vi "DPT Panel RMC Calculator.vi"(0 "Scale Com Port":refnum<visa-resource-name>="COM1", 5 "Bone Dry Weight (lbs)":T2 format="%.3f", 7 "Read Scale Weight":bool, 11 "Error In":errorcluster) -> (6 "DPT IMC Data Out":T3={"Measured IMC (lbs)"=7.0, "Actual Initial RMC (%)"=7.0, "RMC (Desired %)"=100.0, "Bone Dry Wt(lbs)"=7.0, "Tolerance(%)"=5.0, "Actual Final RMC (%)"=7.0, "CEF (lbf/kWh)"=0.0, "Minimum Weight (lbf)"=0.0, "Average Weight (lbf)"=0.0, "Maximum Weight (lbf)"=0.0, "Measured IMC In Range?"=FALSE, "Moisture Reduction Factor"=55.5, "Field Use Factor"=1.04, "Empty Dryer Cold Weigth"=0.0, "Energy Standard"=enum."D2-Automatic Dryer", "Weight Cloth (lbs)"=0.0, "Relative Moisture Content (%)"=0.0, "Relative Moisture Content - Avg (%)"=0.0} {"Maximum Weight (lbf)" format="%03_6g"; "Average Weight (lbf)" format="%03_6g"; "Minimum Weight (lbf)" format="%03_6g"; "CEF (lbf/kWh)" format="%03_6g"; "Actual Final RMC (%)" format="%03_6g"; "Tolerance(%)" format="%0#_6g"; "Bone Dry Wt(lbs)" format="%03_6g"; "RMC (Desired %)" format="%0#_6g"; "Actual Initial RMC (%)" format="%03_6g"; "Measured IMC (lbs)" format="%0#_6g"}, 15 "Error Out":errorcluster)   [LabVIEW 2016, in "File Setup.lvlib"]
uses:
  File Setup.lvlib
  Type Definition/DPT IMC Data.ctl
  Washer DOE/Type Definitions/DOE Dryer Standard.ctl
  Custom Pallet Controls/Custom Pallet DBL.ctl
  Custom Pallet Controls/Custom Pallet Forward.ctl
panel:
  in  "Complete":T1
  out "Average Weight (lbs)":T2 format="%.3f"
  out "Maximum Weight (lbs)":T2 format="%.3f"
  out "Minimum Weight (lbs)":T2 format="%.3f"
  in  "Relative Moisture Content (Desired)":T2 format="%.3f"
  in  "Tolerance %":T2=5.0 format="%.3f"
  in  "Tab Control":enum32{"Page 1", "Page 2"}(tab)
  out "Actual Relative Moisture Content (%)":T2 format="%.2f"
  in  "Measured Initial Moisture Content (lbs)":T2 format="%.3f"
  # "RMC Calculator"
  # "Calculated Result"
  # "User Input"
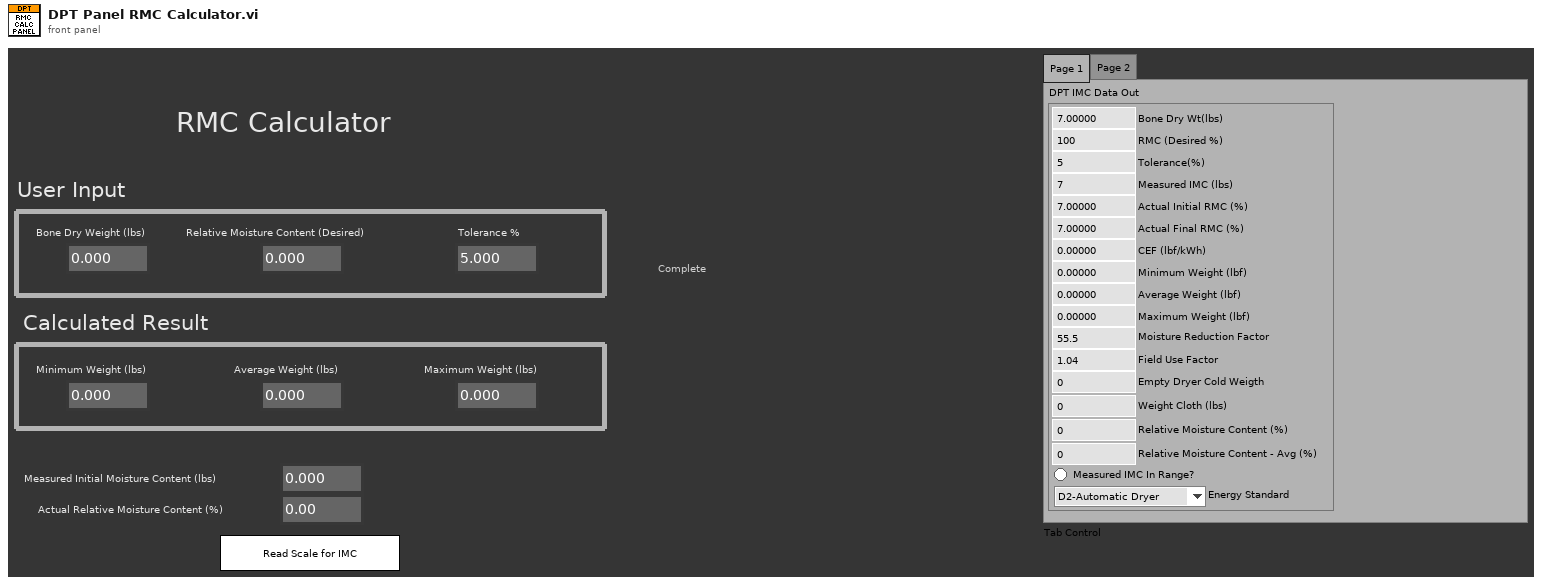
[diagram p1: front panel]
types:
  T1 = typedef "Custom Pallet Forward.ctl" = bool
  T2 = typedef "Custom Pallet DBL.ctl" = dbl
  T3 = typedef "DPT IMC Data.ctl" = cluster{"Measured IMC (lbs)":dbl, "Actual Initial RMC (%)":dbl, "RMC (Desired %)":dbl, "Bone Dry Wt(lbs)":dbl, "Tolerance(%)":dbl, "Actual Final RMC (%)":dbl, "CEF (lbf/kWh)":dbl, "Minimum Weight (lbf)":dbl, "Average Weight (lbf)":dbl, "Maximum Weight (lbf)":dbl, "Measured IMC In Range?":bool, "Moisture Reduction Factor":dbl, "Field Use Factor":dbl, "Empty Dryer Cold Weigth":dbl, "Energy Standard":T4, "Weight Cloth (lbs)":dbl, "Relative Moisture Content (%)":dbl, "Relative Moisture Content - Avg (%)":dbl}
  T4 = typedef "DOE Dryer Standard.ctl" = enum16{"D2-Automatic Dryer", "D2-Timer Dryer", "D1-Automatic Dryer", "D1-Timer Dryer", "Other"}
  T5 = enum32{"invalid app kind", "Development System", "Run Time System", "Student Edition", "Embedded LabVIEW", "Evaluation", "Custom"}
  T6 = enum32{"Invalid", "Standard", "Closed", "Hidden", "Minimized", "Maximized"}
  T7 = cluster{"Core":cluster{"Current VI Reference":refnum<vi>, "Close Panel on Exit?":bool}, "Average Weight (lbs) Show":T2, "Minimum Weight (lbs) Show":T2, "Maximum Weight (lbs) Show":T2, "Scale Com Port":refnum<visa-resource-name>, "DPT IMC Data":T3}
  T8 = cluster{"Current VI Reference":refnum<vi>, "Close Panel on Exit?":bool}
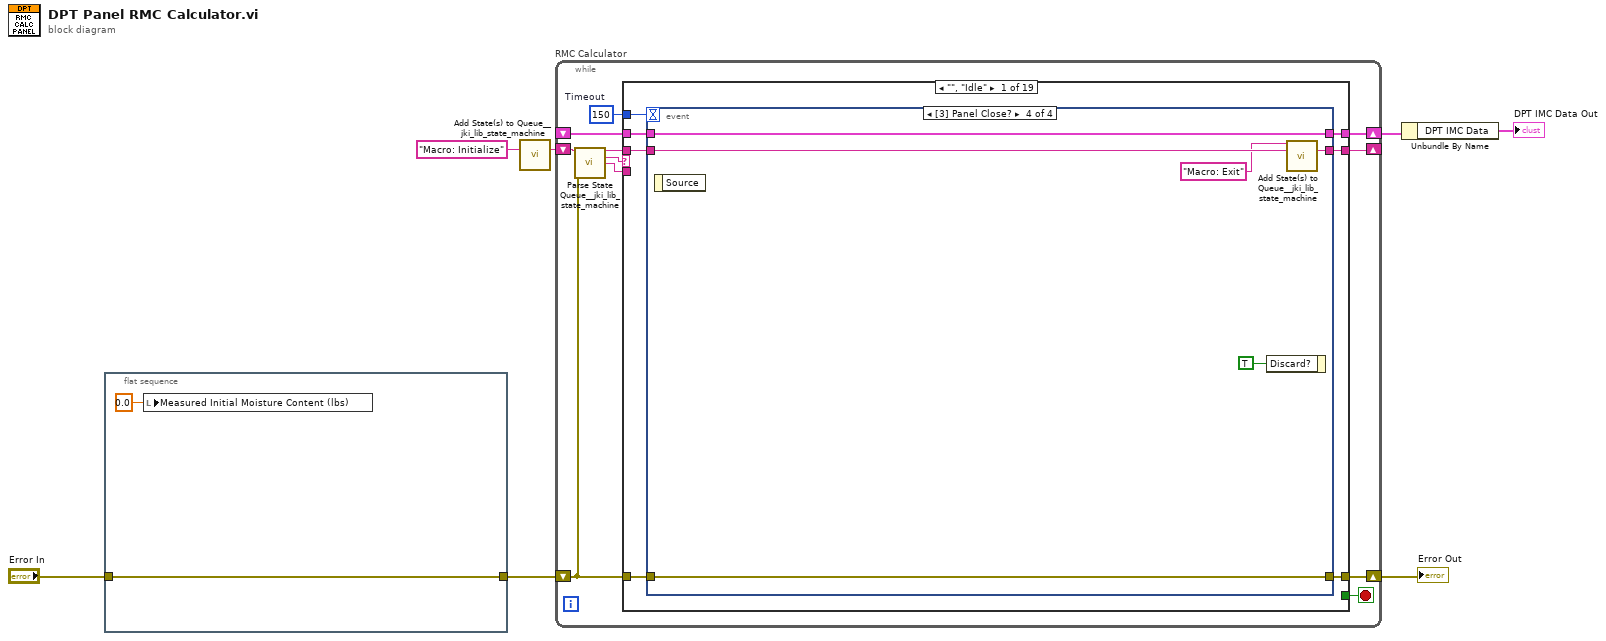
[diagram p0: block diagram]
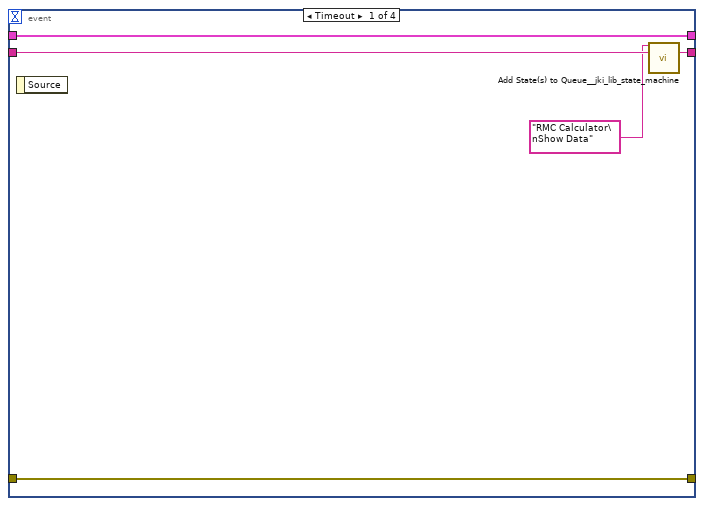
[diagram p2: hidden frame]
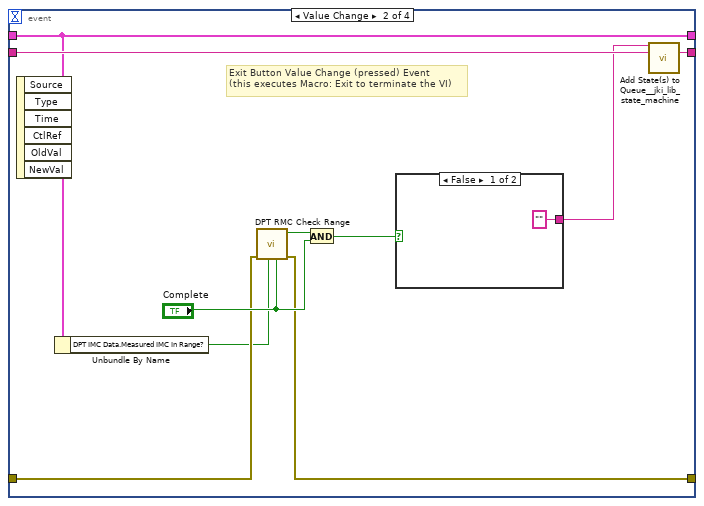
[diagram p3: hidden frame]
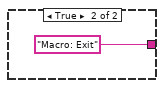
[diagram p4: hidden frame]
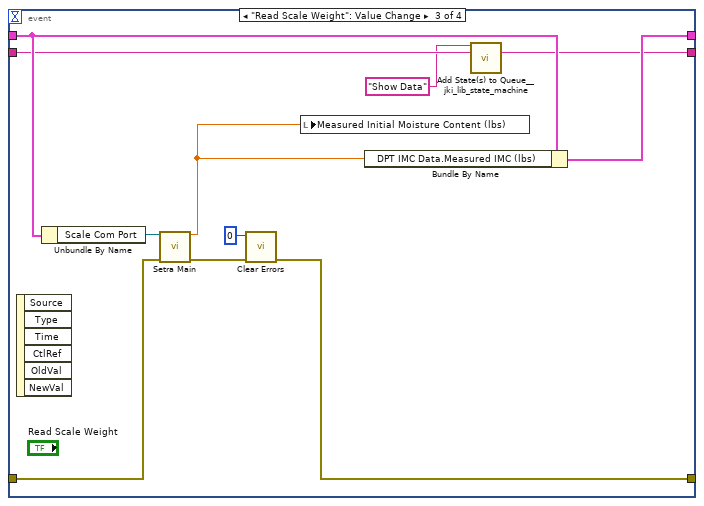
[diagram p5: hidden frame]
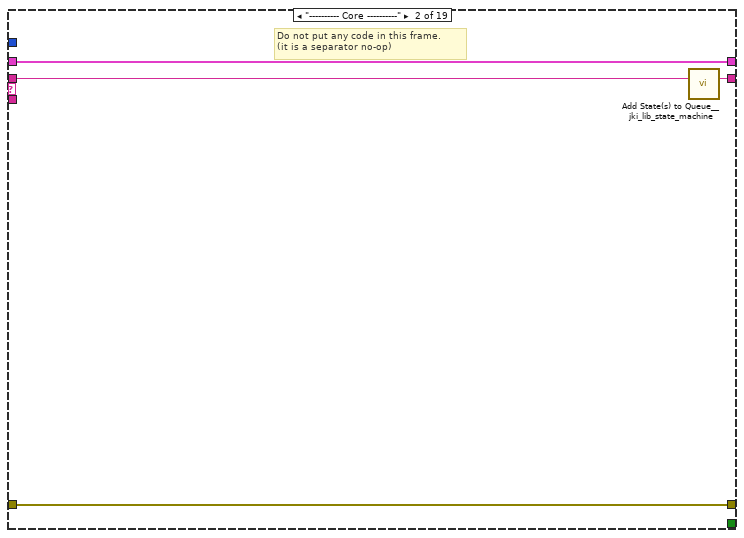
[diagram p6: hidden frame]
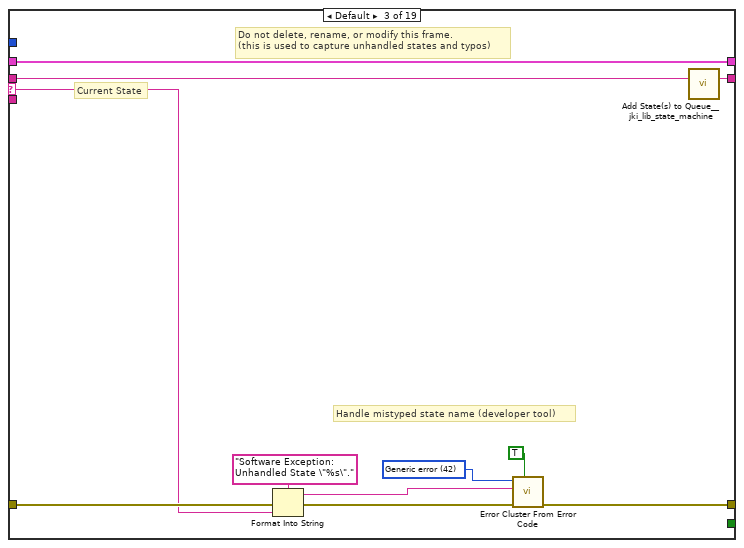
[diagram p7: hidden frame]
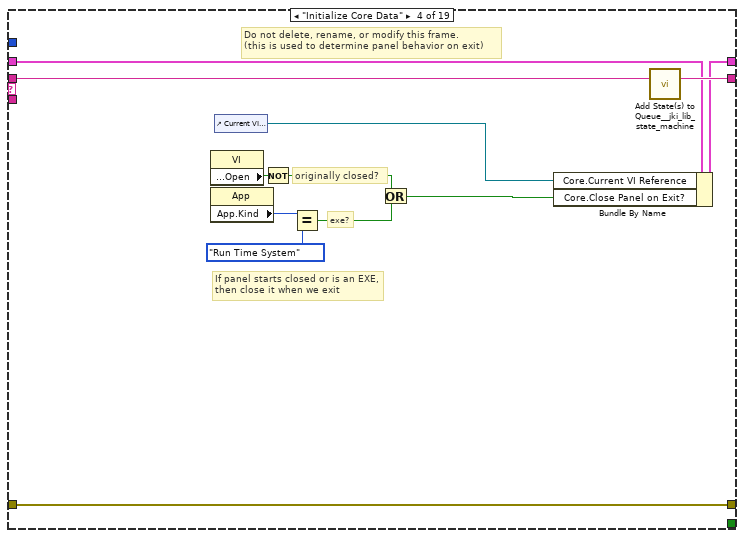
[diagram p8: hidden frame]
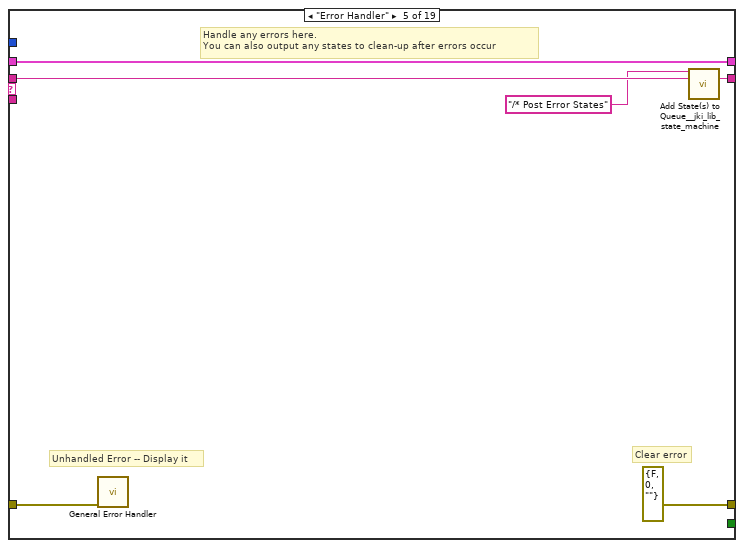
[diagram p9: hidden frame]
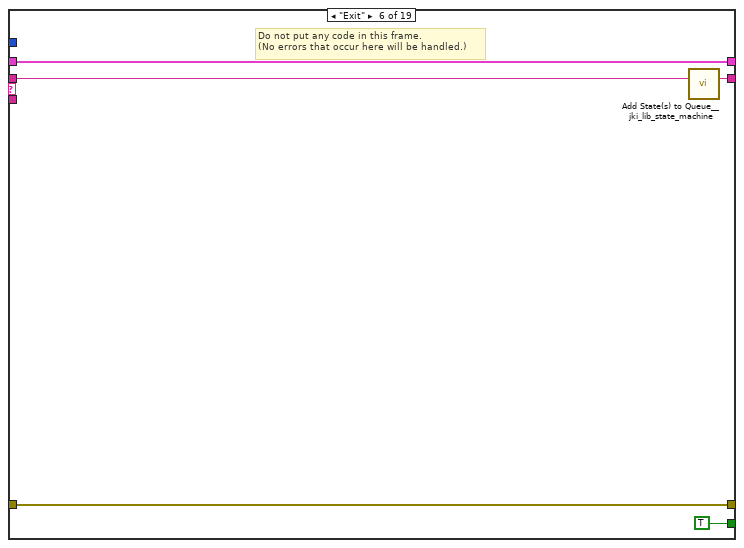
[diagram p10: hidden frame]
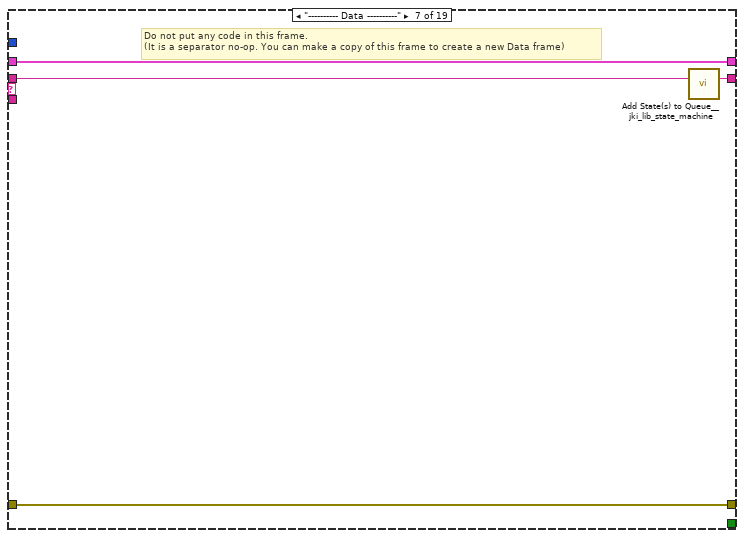
[diagram p11: hidden frame]
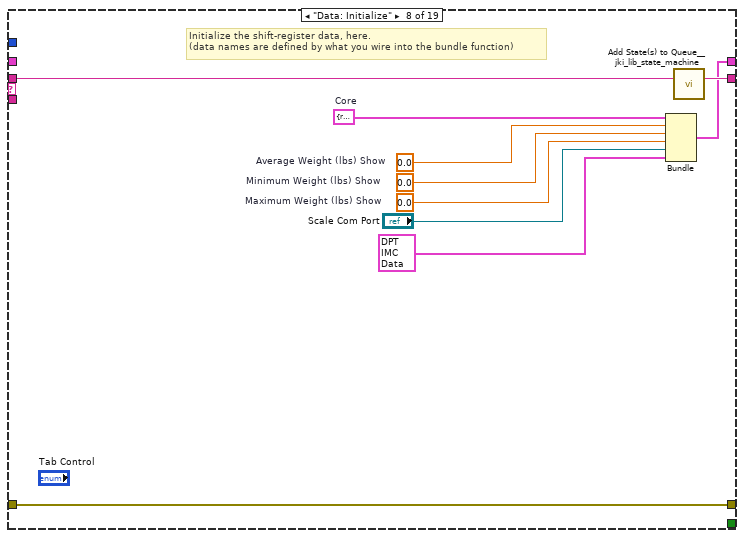
[diagram p12: hidden frame]
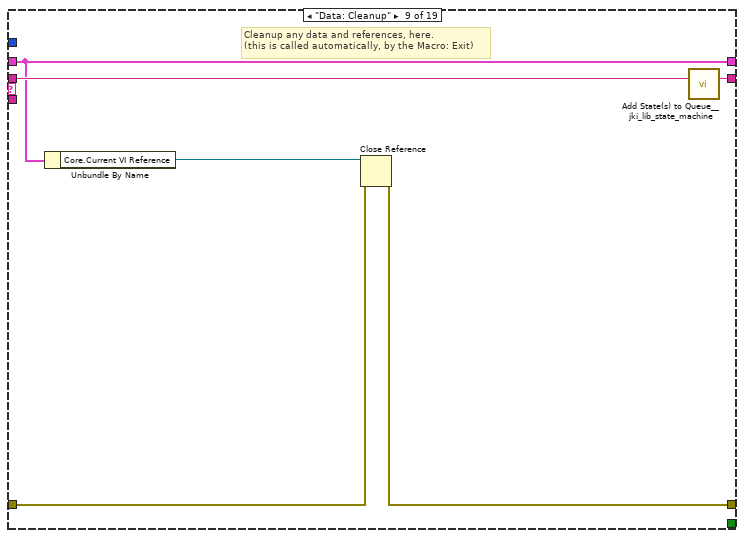
[diagram p13: hidden frame]
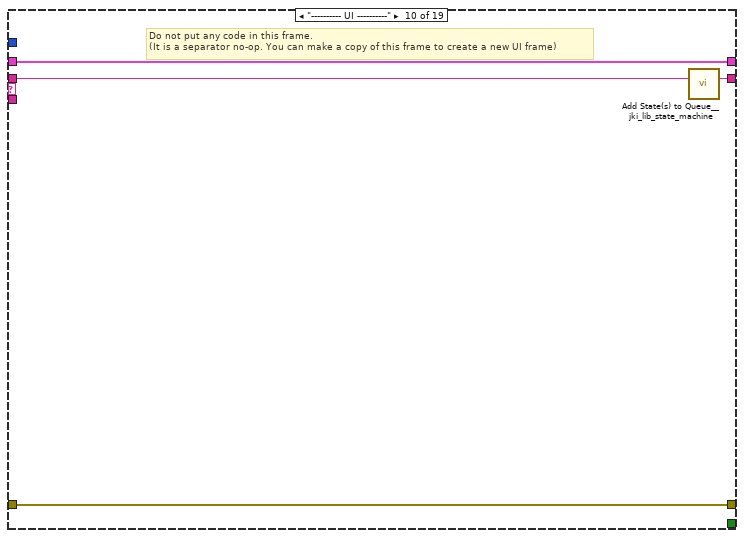
[diagram p14: hidden frame]
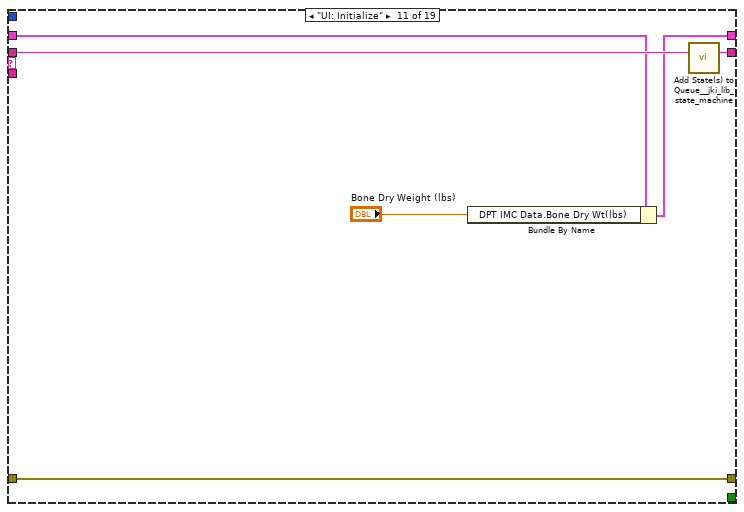
[diagram p15: hidden frame]
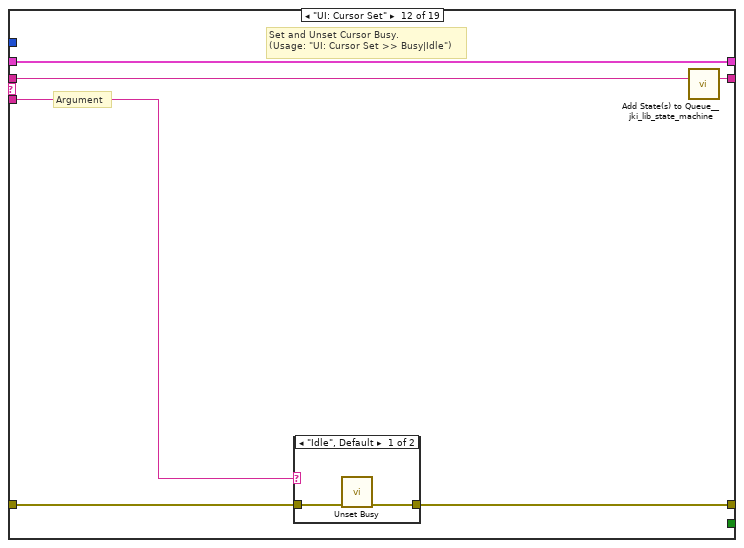
[diagram p16: hidden frame]
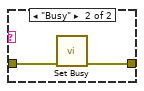
[diagram p17: hidden frame]
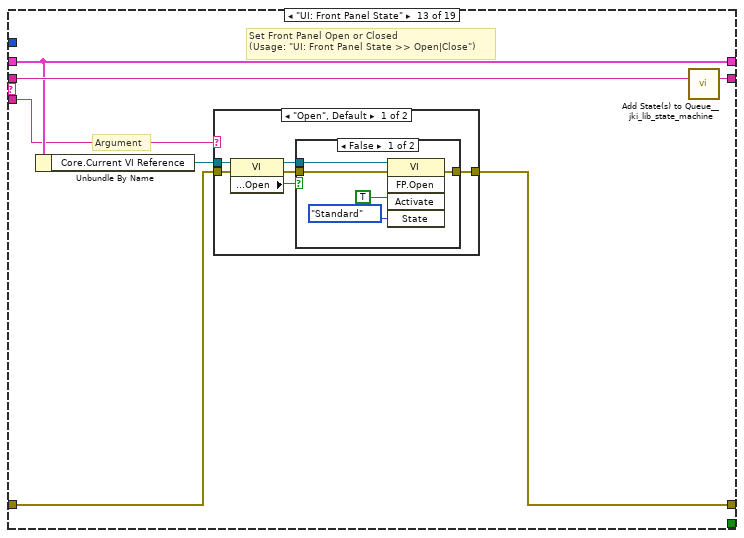
[diagram p18: hidden frame]
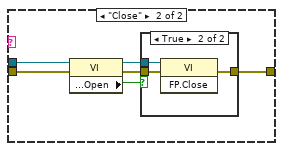
[diagram p20: hidden frame]
diagram:
  n1 = flat-sequence {
    tunnel: "Error In" -> [w8]
    tunnel: [w8] -> w3
    frame #0 {
      n2 = local write "Measured Initial Moisture Content (lbs)"(0.0 ("Measured IMC(Initial Moisture Content)")) -> ()
    }
  }
  n3 = call <vilib>:"Add State(s) to Queue__jki_lib_state_machine.vi"("State(s) in (\"\")"="Macro: Initialize") -> ("States Out"=w7:string)  [unwired: 14 in]
  n4 = while "RMC Calculator" {
    shift-right: [w13] -> w2
    shift-left: _ -> [w12]
    shift-right: [w16] -> w5
    shift-left: w3 -> [w10]
    shift-right: [w15] -> _
    shift-left: w7 -> [w17]
    stop <- w14 stop-if-true
    w11 = 150  # Timeout
    n5 = call <vilib>:"Parse State Queue__jki_lib_state_machine.vi"("State Queue"=w17, "Error In (no error)"=w10) -> ("Remaining States"=w19:string, "Current State"=w20:string, "Arguments"=w18:string)  [unwired: 11 in]
    n6 = case shown="\"\", \"Idle\"" w20 {
      selector: w20 -> [_ _ w66 _ _ _ _ _ _ _ _ _ _ _ _ _ _ _ _]
      tunnel: w19 -> [w27 w65 w70 w88 w94 w99 w103 w113 w119 w123 w129 w135 w146 w172 w177 w187 w191 w199 w209]
      tunnel: w18 -> [_ _ _ _ _ _ _ _ _ _ _ w130 w140 _ _ _ _ _ _]
      tunnel: w12 -> [w25 w62 w68 w79 w91 w97 w100 _ w114 w120 w126 w133 w142 w169 w174 w184 w188 w193 w206]
      tunnel: [w24 w63 w72 w85 errorcluster {"status"=FALSE, "code"=0, "source"=""} ("error out") w96 w101 w110 w115 w121 w127 w131 w143 w170 w175 w185 w189 w197 w207] -> w16
      tunnel: w10 -> [w23 w63 w71 w85 w90 w96 w101 w110 w116 w121 w127 w132 w144 w170 w175 w185 w189 w196 w207]
      tunnel: [w26 w64 w69 w87 w93 w98 w102 w112 w118 w122 w128 w134 w145 w171 w176 w186 w190 w198 w208] -> w15
      tunnel: [_ _ _ _ _ TRUE _ _ _ _ _ _ _ _ _ _ _ _ _] -> w14
      tunnel: [w22 w62 w68 w86 w91 w97 w100 w111 w114 w120 w125 w133 w142 w169 w174 w184 w188 w195 w206] -> w13
      tunnel: w11 -> [w21 _ _ _ _ _ _ _ _ _ _ _ _ _ _ _ _ _ _]
      frame "", "Idle" {
        n7 = event shown="[3] Panel Close?" {
          selector: _ -> [_ _ _ _]
          dyn-events: _ -> [_ _ _ _]
          timeout: w21 -> [_ _ _ _]
          tunnel: w27 -> [w32 w42 w51 w61]
          tunnel: [w31 w41 w50 w60] -> w26
          tunnel: w25 -> [w29 w34 w53 w58]
          tunnel: [w30 w36 w47 w59] -> w24
          tunnel: w23 -> [w30 w37 w55 w59]
          tunnel: [w29 w34 w54 w58] -> w22
          event Timeout {
            n8 = event-data() -> ()  [unwired: 1 in, 1 out]
            n9 = call <vilib>:"Add State(s) to Queue__jki_lib_state_machine.vi"("State(s) in Front (\"\")"="RMC Calculator\nShow Data", "State(s) in (\"\")"=w32) -> ("States Out"=w31:string)  [unwired: 13 in]
          }
          event Value Change {
            # "Exit Button Value Change (pressed) Event\n(this executes Macro: Exit to terminate the VI)"
            n10 = event-data() -> ()  [unwired: 1 in, 6 out]
            n11 = Unbundle By Name(w34) -> ("DPT IMC Data.Measured IMC In Range?"=w33:bool)
            n12 = call "DPT RMC Check Range.vi"("Complete"="Complete", "In Range?"=w33, "Error In"=w37) -> ("Error Out"=w36:errorcluster, "End"=w38:bool)  [unwired: 7 in]
            n13 = And(x=w38, y="Complete") -> (x .and. y?=w35:T1)
            n14 = case shown="False" w35 {
              tunnel: ["" "Macro: Exit"] -> w40
              frame False {
              }
              frame True {
              }
            }
            n15 = call <vilib>:"Add State(s) to Queue__jki_lib_state_machine.vi"("State(s) in Front (\"\")"=w40, "State(s) in (\"\")"=w42) -> ("States Out"=w41:string)  [unwired: 13 in]
          }
          event "Read Scale Weight": Value Change {
            n16 = event-data() -> ()  [unwired: 1 in, 6 out]
            n17 = Unbundle By Name(w53) -> ("Scale Com Port"=w52:refnum<visa-resource-name>)
            n18 = call "Setra Main.vi"("VISA resource name"=w52, "Error In"=w55) -> ("Weight Output"=w45:dbl, "Error Out"=w48:errorcluster)  [unwired: 11 in, 1 out]
            n19 = call <vilib>:"Clear Errors.vi"("error in (no error)"=w48, "specific error code to clear (0: all)"=0) -> ("error out"=w47:errorcluster)  [unwired: 4 in, 1 out]
            n20 = local write "Measured Initial Moisture Content (lbs)"(w45) -> ()
            n21 = Bundle By Name(cluster=w53, "DPT IMC Data.Measured IMC (lbs)"=w45) -> (w54:T7)
            n22 = call <vilib>:"Add State(s) to Queue__jki_lib_state_machine.vi"("State(s) in Front (\"\")"="Show Data", "State(s) in (\"\")"=w51) -> ("States Out"=w50:string)  [unwired: 13 in]
          }
          event Panel Close? {
            n23 = event-data() -> ()  [unwired: 1 in, 1 out]
            n24 = event-data("Discard?"=TRUE) -> ()  [unwired: 1 in, 1 out]
            n25 = call <vilib>:"Add State(s) to Queue__jki_lib_state_machine.vi"("State(s) in Front (\"\")"="Macro: Exit", "State(s) in (\"\")"=w61) -> ("States Out"=w60:string)  [unwired: 13 in]
          }
        }
      }
      frame "---------- Core ----------" {
        # "Do not put any code in this frame.\n(it is a separator no-op)"
        n26 = call <vilib>:"Add State(s) to Queue__jki_lib_state_machine.vi"("State(s) in (\"\")"=w65) -> ("States Out"=w64:string)  [unwired: 14 in]
      }
      frame Default {
        w75 = 42 items=["No error", "Argument error", "Memory is full", "Out of zone", "End of file", "File already open", "Generic file I/O error", "File not found", "File permission error", "Disk is full", "Duplicate path", "Too many files open", "System feature not enabled", "Resource file not found", "Cannot add resource", "Resource not found", "Image not found", "Image memory error", "Pen does not exist", "Config type invalid", "Config token not found", "Config parse error", "Config memory error", "Bad external code format", "Bad external code offset", "External code not present", "Null window", "Destroy window error", "Null menu", "Print aborted", "Bad print record", "Print driver error", "Windows error during printing", "Memory error during printing", "Print dialog error", "Generic print error", "Invalid device refnum", "Device not found", "Device parameter error", "Device unit error", "Cannot open device", "Device call aborted", "Generic error", "Cancelled by user", "Object ID too low", "Object ID too high", "Object not in heap", "Unknown heap", "Unknown object (invalid DefProc)", "Unknown object (DefProc not in table)", "Message out of range", "Invalid (null) method", "Unknown message", "Manager call not supported", "Bad address", "Network operation in progress", "Network operation timed out", "Connection is busy", "Network attribute not supported", "Network error", "Address in use", "System out of memory", "Connection aborted", "Connection refused", "Not connected", "Already connected", "Connection closed", "Initialization error (interapplication manager)", "Bad occurrence", "Wait on unbound occurrence handler", "Occurrence queue overflow", "Datalog type conflict", "Unused", "Unrecognized type (interapplication manager)", "Memory corrupt", "Failed to make temporary DLL", "Old CIN version", "Drag socket not found", "Failed to load drop-object", "Failed to register OLE object", "Failed to release OLE object", "Format specifier type mismatch", "Unknown format specifier", "Too few format specifiers", "Too many format specifiers", "Scan failed", "Newer CIN version", "Error converting to variant", "Runtime menu error", "Password tampered", "Variant attribute not found", "Incompatible variant data type", "Event data is not available", "Event Store is not present", "Occurrence is not found", "Event Queue is not created", "Event info is not available", "Refnum passed is NULL", "Error retrieving Class GUID", "Error retrieving CoClass GUID", "Error retrieving TypeLib GUID.", "Bad built application magic bytes.", "Specific driver is different from the specific driver associated with the Logical Name.", "There is no session opened to the class driver.", "Max Error", "MAX - Error with config objects", "MAX - Error loading configuration", "MAX - Group not supported"]
        # "Current State"
        # "Do not delete, rename, or modify this frame.\n(this is used to capture unhandled states and typos)"
        # "Handle mistyped state name (developer tool)"
        n27 = Format Into String(format string="Software Exception: Unhandled State \"%s\"." ("message"), error in=w71, w66) -> (resulting string=w74:string, error out=w73:errorcluster)  [unwired: 1 in]
        n28 = call <vilib>:"Error Cluster From Error Code.vi"("show call chain? (False)"=TRUE, "error in (no error)"=w73, "error message (\"\")"=w74, "error code (0)"=w75) -> ("error out"=w72:errorcluster)  [unwired: 5 in]
        n29 = call <vilib>:"Add State(s) to Queue__jki_lib_state_machine.vi"("State(s) in (\"\")"=w70) -> ("States Out"=w69:string)  [unwired: 14 in]
      }
      frame "Initialize Core Data" {
        # "Do not delete, rename, or modify this frame.\n(this is used to determine panel behavior on exit)"
        # "originally closed?"
        # "exe?"
        # "If panel starts closed or is an EXE, then close it when we exit"
        n30 = property class="VI"() -> ("Front Panel.Open"=w84:bool)  [unwired: 2 in, 2 out]
        n31 = property class="App"() -> ("App.Kind"=w83:T5)  [unwired: 2 in, 2 out]
        n32 = control-ref of="Current VI Reference"() -> (w77:refnum<vi>)
        n33 = Not(x=w84) -> (.not. x?=w81:bool)
        n34 = Equal?(x=w83, y=T5."Run Time System" ("Application:Kind")) -> (x = y?=w80:bool)
        n35 = Or(x=w81, y=w80) -> (x .or. y?=w78:bool)
        n36 = Bundle By Name(cluster=w79, "Core.Current VI Reference"=w77, "Core.Close Panel on Exit?"=w78) -> (w86:T7)
        n37 = call <vilib>:"Add State(s) to Queue__jki_lib_state_machine.vi"("State(s) in (\"\")"=w88) -> ("States Out"=w87:string)  [unwired: 14 in]
      }
      frame "Error Handler" {
        # "Unhandled Error -- Display it"
        # "Handle any errors here.\nYou can also output any states to clean-up after errors occur"
        # "Clear error"
        n38 = call <vilib>:"General Error Handler.vi"("error in (no error)"=w90) -> ()  [unwired: 10 in, 5 out]
        n39 = call <vilib>:"Add State(s) to Queue__jki_lib_state_machine.vi"("State(s) in Front (\"\")"="/* Post Error States", "State(s) in (\"\")"=w94) -> ("States Out"=w93:string)  [unwired: 13 in]
      }
      frame "Exit" {
        # "Do not put any code in this frame.\n(No errors that occur here will be handled.)"
        n40 = call <vilib>:"Add State(s) to Queue__jki_lib_state_machine.vi"("State(s) in (\"\")"=w99) -> ("States Out"=w98:string)  [unwired: 14 in]
      }
      frame "---------- Data ----------" {
        # "Do not put any code in this frame.\n(It is a separator no-op. You can make a copy of this frame to create a new Data frame)"
        n41 = call <vilib>:"Add State(s) to Queue__jki_lib_state_machine.vi"("State(s) in (\"\")"=w103) -> ("States Out"=w102:string)  [unwired: 14 in]
      }
      frame "Data: Initialize" {
        w106 = T2 0.0  # Maximum Weight (lbs) Show
        w107 = T2 0.0  # Minimum Weight (lbs) Show
        w108 = T2 0.0  # Average Weight (lbs) Show
        w109 = T8 {"Current VI Reference"=refnum, "Close Panel on Exit?"=FALSE}  # Core
        # "Initialize the shift-register data, here.\n(data names are defined by what you wire into the bundle function)"
        n42 = Bundle("Core"=w109, "Average Weight (lbs) Show"=w108, "Minimum Weight (lbs) Show"=w107, "Maximum Weight (lbs) Show"=w106, "Scale Com Port"="Scale Com Port", "DPT IMC Data"=T3 {"Measured IMC (lbs)"=0.0, "Actual Initial RMC (%)"=0.0, "RMC (Desired %)"=0.0, "Bone Dry Wt(lbs)"=0.0, "Tolerance(%)"=5.0, "Actual Final RMC (%)"=7.0, "CEF (lbf/kWh)"=0.0, "Minimum Weight (lbf)"=0.0, "Average Weight (lbf)"=0.0, "Maximum Weight (lbf)"=0.0, "Measured IMC In Range?"=FALSE, "Moisture Reduction Factor"=55.5, "Field Use Factor"=1.04, "Empty Dryer Cold Weigth"=0.0, "Energy Standard"=enum."D2-Automatic Dryer", "Weight Cloth (lbs)"=0.0, "Relative Moisture Content (%)"=0.0, "Relative Moisture Content - Avg (%)"=0.0}) -> (w111:T7)  [unwired: 1 in]
        n43 = call <vilib>:"Add State(s) to Queue__jki_lib_state_machine.vi"("State(s) in (\"\")"=w113) -> ("States Out"=w112:string)  [unwired: 14 in]
      }
      frame "Data: Cleanup" {
        # "Cleanup any data and references, here.\n(this is called automatically, by the Macro: Exit)"
        n44 = Unbundle By Name(w114) -> ("Core.Current VI Reference"=w117:refnum<vi>)
        n45 = Close Reference(reference=w117, error in (no error)=w116) -> (error out=w115:errorcluster)
        n46 = call <vilib>:"Add State(s) to Queue__jki_lib_state_machine.vi"("State(s) in (\"\")"=w119) -> ("States Out"=w118:string)  [unwired: 14 in]
      }
      frame "---------- UI ----------" {
        # "Do not put any code in this frame.\n(It is a separator no-op. You can make a copy of this frame to create a new UI frame)"
        n47 = call <vilib>:"Add State(s) to Queue__jki_lib_state_machine.vi"("State(s) in (\"\")"=w123) -> ("States Out"=w122:string)  [unwired: 14 in]
      }
      frame "UI: Initialize" {
        n48 = Bundle By Name(cluster=w126, "DPT IMC Data.Bone Dry Wt(lbs)"="Bone Dry Weight (lbs)") -> (w125:T7)
        n49 = call <vilib>:"Add State(s) to Queue__jki_lib_state_machine.vi"("State(s) in (\"\")"=w129) -> ("States Out"=w128:string)  [unwired: 14 in]
      }
      frame "UI: Cursor Set" {
        # "Argument"
        # "Set and Unset Cursor Busy.\n(Usage: \"UI: Cursor Set >> Busy|Idle\")"
        n50 = case shown="\"Idle\", Default" w130 {
          tunnel: w132 -> [w137 w139]
          tunnel: [w136 w138] -> w131
          frame "Idle", Default {
            n51 = call <vilib>:"Unset Busy.vi"("error in (no error)"=w137) -> ("error out"=w136:errorcluster)  [unwired: 10 in]
          }
          frame "Busy" {
            n52 = call <vilib>:"Set Busy.vi"("error in (no error)"=w139) -> ("error out"=w138:errorcluster)  [unwired: 9 in, 1 out]
          }
        }
        n53 = call <vilib>:"Add State(s) to Queue__jki_lib_state_machine.vi"("State(s) in (\"\")"=w135) -> ("States Out"=w134:string)  [unwired: 14 in]
      }
      frame "UI: Front Panel State" {
        # "Argument"
        # "Set Front Panel Open or Closed\n(Usage: \"UI: Front Panel State >> Open|Close\")"
        n54 = Unbundle By Name(w142) -> ("Core.Current VI Reference"=w141:refnum<vi>)
        n55 = case shown="\"Open\", Default" w140 {
          tunnel: w144 -> [w150 w163]
          tunnel: [w152 w164] -> w143
          tunnel: w141 -> [w151 w161]
          frame "Open", Default {
            n56 = property class="VI"(reference=w151, error in=w150) -> (reference out=w148:refnum<vi>, error out=w149:errorcluster, "Front Panel.Open"=w147:bool)
            n57 = case shown="False" w147 {
              tunnel: [w155 w158] -> w152
              tunnel: w149 -> [w154 w158]
              tunnel: w148 -> [w153 _]
              frame False {
                n58 = invoke class="VI" method="FP.Open"(reference=w153, error in=w154, "Activate"=TRUE, "State"=T6."Standard") -> (error out=w155:errorcluster)  [unwired: 1 in, 4 out]
              }
              frame True {
              }
            }
          }
          frame "Close" {
            n59 = property class="VI"(reference=w161, error in=w163) -> (reference out=w160:refnum<vi>, error out=w162:errorcluster, "Front Panel.Open"=w159:bool)
            n60 = case shown="True" w159 {
              tunnel: [w165 w168] -> w164
              tunnel: w162 -> [w165 w167]
              tunnel: w160 -> [_ w166]
              frame False {
              }
              frame True {
                n61 = invoke class="VI" method="FP.Close"(reference=w166, error in=w167) -> (error out=w168:errorcluster)  [unwired: 1 in, 2 out]
              }
            }
          }
        }
        n62 = call <vilib>:"Add State(s) to Queue__jki_lib_state_machine.vi"("State(s) in (\"\")"=w146) -> ("States Out"=w145:string)  [unwired: 14 in]
      }
      frame "---------- Macro ----------" {
        # "Do not put any code in this frame.\n(It is a separator no-op. You can make a copy of this frame to create a new Macro frame)"
        n63 = call <vilib>:"Add State(s) to Queue__jki_lib_state_machine.vi"("State(s) in (\"\")"=w172) -> ("States Out"=w171:string)  [unwired: 14 in]
      }
      frame "Macro: Initialize" {
        w173 = "Data: Initialize\nInitialize Core Data\nUI: Initialize\nUI: Front Panel State >> Open"  # Data: Initialize Initialize Core Data UI: Initialize UI: Front Panel State >> Open
        # "Initialization Macro\n(This is called once, when the VI starts)"
        n64 = call <vilib>:"Add State(s) to Queue__jki_lib_state_machine.vi"("State(s) in Front (\"\")"=w173, "State(s) in (\"\")"=w177) -> ("States Out"=w176:string)  [unwired: 13 in]
      }
      frame "Macro: Exit" {
        # "Exit Macro\n(This is called once, when the VI exits)"
        n65 = Unbundle By Name(w184) -> ("Core.Close Panel on Exit?"=w183:bool)
        n66 = Select(t="UI: Front Panel State >> Close", s=w183, f="") -> (s? t:f=w180:string)
        n67 = call <vilib>:"Add State(s) to Queue__jki_lib_state_machine.vi"("State(s) in (\"\")"=w180, "State(s) at Back (\"\")"="Data: Cleanup\nExit") -> ("States Out"=w178:string)  [unwired: 13 in]
        n68 = call <vilib>:"Add State(s) to Queue__jki_lib_state_machine.vi"("State(s) in Front (\"\")"=w178, "State(s) in (\"\")"=w187) -> ("States Out"=w186:string)  [unwired: 13 in]
      }
      frame "---------- New Category ----------" {
        # "Template Separator\n(You can make a copy of, or modify, this frame)"
        n69 = call <vilib>:"Add State(s) to Queue__jki_lib_state_machine.vi"("State(s) in (\"\")"=w191) -> ("States Out"=w190:string)  [unwired: 14 in]
      }
      frame "RMC Calculator" {
        n70 = Unbundle By Name(w193) -> ("DPT IMC Data"=w192:T3)
        n71 = call "Save File DPT RMC Calculations.vi"("Dryer IMC Data Input"=w192, "Error In"=w196) -> ("Dryer IMC Data Output"=w194:T3, "Error Out"=w197:errorcluster)  [unwired: 16 in]
        n72 = Bundle By Name(cluster=w193, "DPT IMC Data"=w194) -> (w195:T7)
        n73 = call <vilib>:"Add State(s) to Queue__jki_lib_state_machine.vi"("State(s) in (\"\")"=w199) -> ("States Out"=w198:string)  [unwired: 14 in]
      }
      frame "Show Data" {
        n74 = Unbundle By Name(w206) -> ("Average Weight (lbs) Show"=→"Average Weight (lbs)":T2, "DPT IMC Data.Bone Dry Wt(lbs)"=w204:dbl, "DPT IMC Data.Measured IMC (lbs)"=w203:dbl, "Minimum Weight (lbs) Show"=→"Minimum Weight (lbs)":T2, "DPT IMC Data.Actual Initial RMC (%)"=→"Actual Relative Moisture Content (%)":dbl, "Maximum Weight (lbs) Show"=→"Maximum Weight (lbs)":T2)
        n75 = local write "Bone Dry Weight (lbs)"(w204) -> ()
        n76 = local write "Measured Initial Moisture Content (lbs)"(w203) -> ()
        n77 = call <vilib>:"Add State(s) to Queue__jki_lib_state_machine.vi"("State(s) in (\"\")"=w209) -> ("States Out"=w208:string)  [unwired: 14 in]
      }
    }
  }
  "Error Out" <- w5
  n78 = Unbundle By Name(w2) -> ("DPT IMC Data"=→"DPT IMC Data Out":T3)
